vi "Display in Grid.vi"(8 "error in (no error)":errorcluster, 10 "ViewableActor":refnum<class "Message Enqueuer.lvclass">, 11 "DemoMain in":refnum<class "DemoMain.lvclass">) -> (0 "error out":errorcluster, 3 "DemoMain out":refnum<class "DemoMain.lvclass">)   [LabVIEW 2012, in "Win8uiDemo.lvlib" / "DemoMain.lvclass"]
uses:
  DemoMain.lvclass
  <vilib>/ActorFramework/Message Enqueuer/Message Enqueuer.lvclass
  Win8uiFramework/MainController.lvclass/MainController.ctl
  SubPanel Grid View Messages/Display ViewableActor Msg/Display ViewableActor Msg.lvclass/Display ViewableActor Msg.ctl
  <vilib>/ActorFramework/Message Enqueuer/Message Enqueuer.lvclass/Message Enqueuer.ctl
  Win8uiFramework/Read MainPane Enqueuer.vi
  <vilib>/ActorFramework/Message Enqueuer/Enqueue.vi
  <vilib>/ActorFramework/Message Priority Queue/Priority Enqueue.vi
  SubPanel Grid View Messages/Display ViewableActor Msg/Display ViewableActor Msg.lvclass
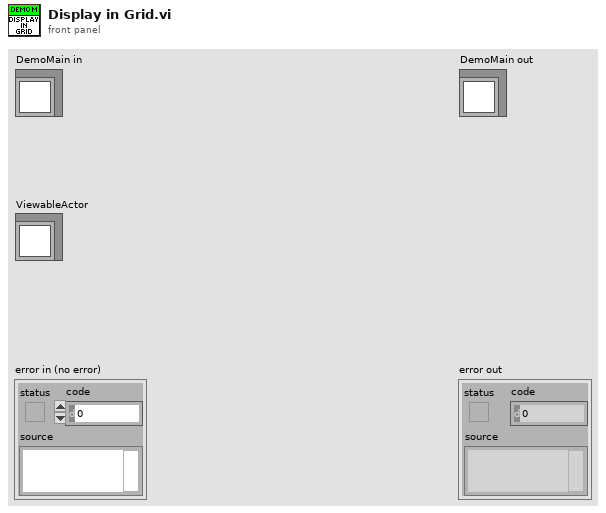
[diagram p1: front panel]
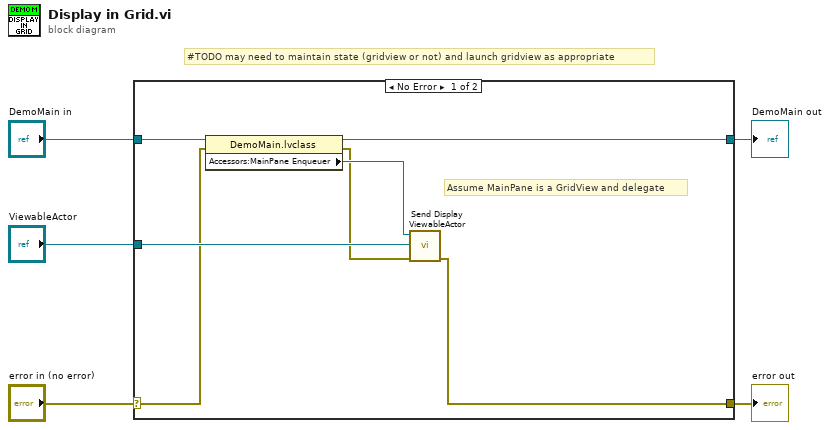
[diagram p0: block diagram]
diagram:
  # "#TODO may need to maintain state (gridview or not) and launch gridview as appropriate"
  n1 = case shown="No Error" "error in (no error)" {
    selector: "error in (no error)" -> [w7 w14]
    tunnel: [w6 w14] -> w4
    tunnel: [w11 w13] -> w2
    tunnel: "DemoMain in" -> [w12 w13]
    tunnel: "ViewableActor" -> [w9 _]
    frame No Error {
      # "Assume MainPane is a GridView and delegate"
      n2 = property class="DemoMain.lvclass"(reference=w12, error in=w7) -> (reference out=w11:refnum<class "DemoMain.lvclass">, error out=w8:errorcluster, "Accessors:MainPane Enqueuer"=w10:refnum<class "Message Enqueuer.lvclass">)
      n3 = call "Send Display ViewableActor.vi"("error in (no error)"=w8, "ViewableActor"=w9, "Message Enqueuer"=w10) -> ("error out"=w6:errorcluster)  [unwired: 7 in, 1 out]
    }
    frame Error {
    }
  }
  "error out" <- w4
  "DemoMain out" <- w2
